vi "Write voltage.vi"(8 "error in (no error)":errorcluster, 10 "voltage":sgl, 11 "Product-B in":refnum<class "Product-B.lvclass">) -> (0 "error out":errorcluster, 3 "Product-B out":refnum<class "Product-B.lvclass">)   [LabVIEW 2018, in "Product-B.lvclass"]
uses:
  Product-B.lvclass
  Product-B.lvclass/Product-B.ctl
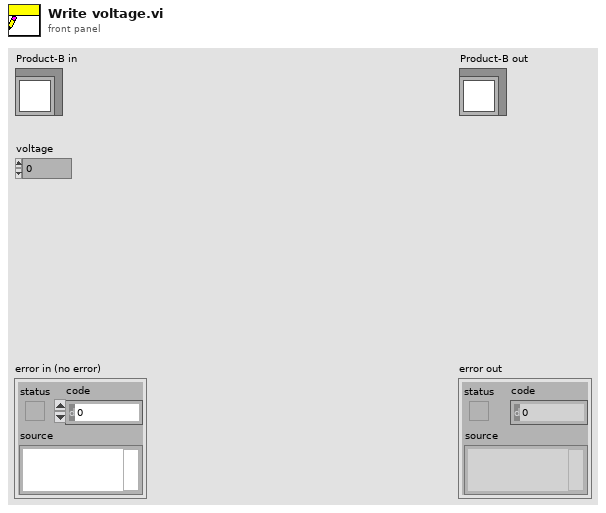
[diagram p1: front panel]
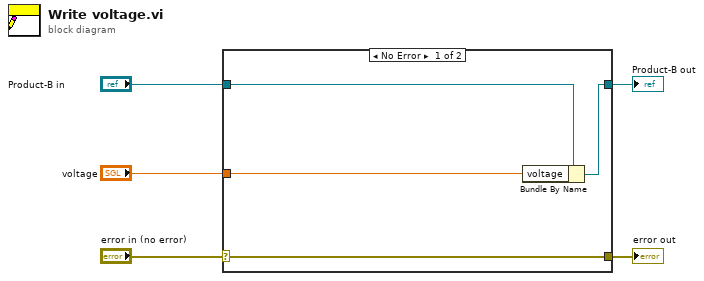
[diagram p0: block diagram]
diagram:
  n1 = case shown="No Error" "error in (no error)" {
    selector: "error in (no error)" -> [w9 w10]
    tunnel: [w9 w10] -> w4
    tunnel: [w7 w11] -> w2
    tunnel: "Product-B in" -> [w8 w11]
    tunnel: "voltage" -> [w6 _]
    frame No Error {
      n2 = Bundle By Name(cluster=w8, "voltage"=w6) -> (w7:refnum<class "Product-B.lvclass">)
    }
    frame Error {
    }
  }
  "error out" <- w4
  "Product-B out" <- w2
